vi "BoatUnderCloudTest.vi"(1 "HDG 2":dbl, 2 "HDG":dbl, 3 "Y 2":dbl, 4 "X 2":dbl, 5 "X":dbl, 6 "Y":dbl) -> (0 "Is the boat \nunder clouds?":bool)   [LabVIEW 2012]
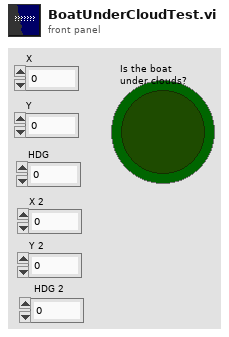
[diagram p1: front panel]
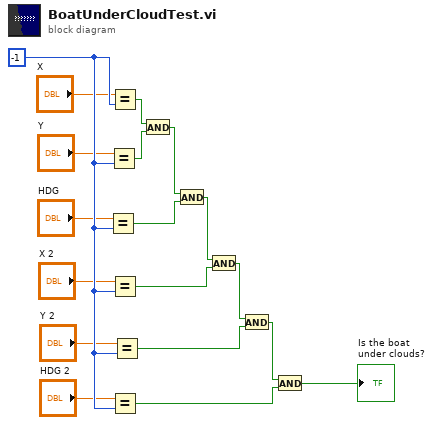
[diagram p0: block diagram]
diagram:
  w18 = -1
  n1 = Equal?(x="HDG", y=w18) -> (x = y?=w9:bool)
  n2 = Equal?(x="Y", y=w18) -> (x = y?=w10:bool)
  n3 = Equal?(x="X", y=w18) -> (x = y?=w11:bool)
  n4 = Equal?(x="X 2", y=w18) -> (x = y?=w6:bool)
  n5 = Equal?(x="HDG 2", y=w18) -> (x = y?=w2:bool)
  n6 = Equal?(x="Y 2", y=w18) -> (x = y?=w4:bool)
  n7 = And(x=w11, y=w10) -> (x .and. y?=w8:bool)
  n8 = And(x=w8, y=w9) -> (x .and. y?=w7:bool)
  n9 = And(x=w7, y=w6) -> (x .and. y?=w5:bool)
  n10 = And(x=w5, y=w4) -> (x .and. y?=w3:bool)
  n11 = And(x=w3, y=w2) -> (x .and. y?=→"Is the boat \nunder clouds?":bool)
